vi "svmdense_train.vi"(8 "error in (no error)":errorcluster, 10 "Parameters":T2, 11 "Problem":T5) -> (0 "error out":errorcluster, 3 "Model":T1)   [LabVIEW 2014]
uses:
  LibSVM Sparse/Wrapper API/Controls/svm_parameter.ctl
  LibSVM Sparse/Wrapper API/Controls/svm_type.ctl
  LibSVM Sparse/Wrapper API/Controls/svm_kernel_type.ctl
  Controls/svmdense_problem.ctl
  Controls/svmdense_node.ctl
  Controls/svmdense_model.ctl
  bin/x64/LabVIEW-libsvm-dense.dll
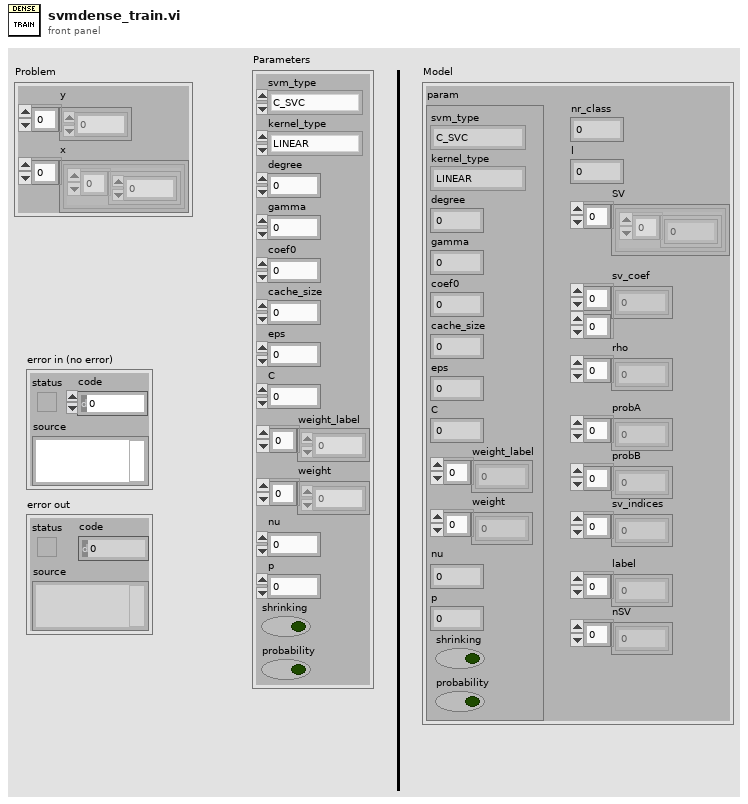
[diagram p1: front panel]
types:
  T1 = typedef "svmdense_model.ctl" = cluster{"param":T2, "nr_class":i32, "l":i32, "SV":cluster{"Array":dbl[]}[], "sv_coef":dbl[][], "rho":dbl[], "probA":dbl[], "probB":dbl[], "sv_indices":i32[], "label":i32[], "nSV":i32[]}
  T2 = typedef "svm_parameter.ctl" = cluster{"svm_type":T3, "kernel_type":T4, "degree":i32, "gamma":dbl, "coef0":dbl, "cache_size":dbl, "eps":dbl, "C":dbl, "weight_label":i32[], "weight":dbl[], "nu":dbl, "p":dbl, "shrinking":bool, "probability":bool}
  T3 = typedef "svm_type.ctl" = enum32{"C_SVC", "NU_SVC", "ONE_CLASS", "EPSILON_SVR", "NU_SVR"}
  T4 = typedef "svm_kernel_type.ctl" = enum32{"LINEAR", "POLY", "RBF", "SIGMOID", "PRECOMPUTED"}
  T5 = typedef "svmdense_problem.ctl" = cluster{"y":dbl[], "x":T6[]}
  T6 = typedef "svmdense_node.ctl" = cluster{"x":dbl[]}
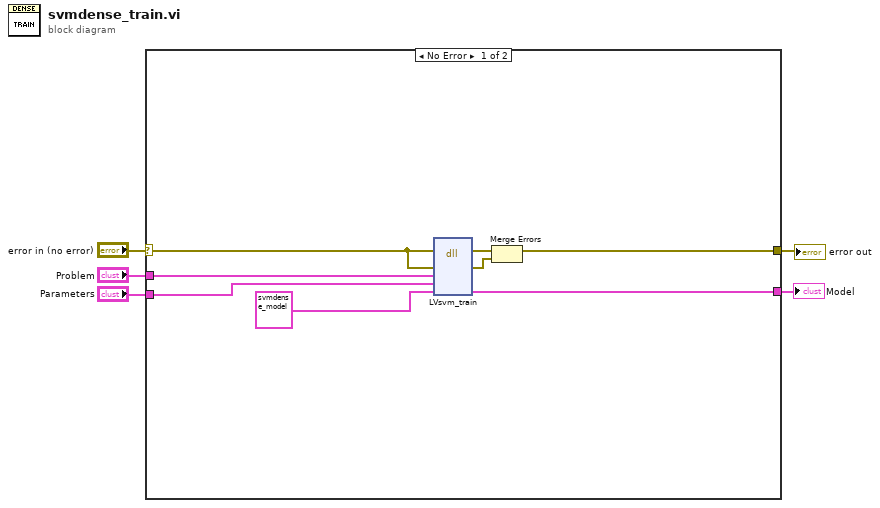
[diagram p0: block diagram]
diagram:
  n1 = case shown="No Error" "error in (no error)" {
    selector: "error in (no error)" -> [w13 w14]
    tunnel: [w12 w14] -> w5
    tunnel: "Problem" -> [w11 _]
    tunnel: "Parameters" -> [w10 _]
    tunnel: [w9 _] -> w1
    frame No Error {
      n2 = dll-call lib="C:/dev/LabVIEW-libsvm/LabVIEW/bin/x64/LabVIEW-libsvm-dense.dll" fn="LVsvm_train"(error in=w13, "lvErr"=w13, "prob_in"=w11, "param_in"=w10, "model_out"=T1 {"param"={"svm_type"=enum."C_SVC", "kernel_type"=enum."LINEAR", "degree"=0, "gamma"=0.0, "coef0"=0.0, "cache_size"=0.0, "eps"=0.0, "C"=0.0, "weight_label"=[], "weight"=[], "nu"=0.0, "p"=0.0, "shrinking"=FALSE, "probability"=FALSE}, "nr_class"=0, "l"=0, "SV"=[], "sv_coef"=[], "rho"=[], "probA"=[], "probB"=[], "sv_indices"=[], "label"=[], "nSV"=[]} ("Model")) -> (error out=w8:errorcluster, "lvErr"=w7:errorcluster, "model_out"=w9:T1)  [unwired: 5 in, 1 out]
      n3 = Merge Errors(w8, w7) -> (w12:errorcluster)
    }
    frame Error {
    }
  }
  "error out" <- w5
  "Model" <- w1
